vi "Range.vi"(8 "Exponent":dbl=1.0, 9 "End":dbl, 10 "Start":dbl, 11 "Steps":i32) -> (3 "Array":dbl[](array[numeric]))   [LabVIEW 2017]
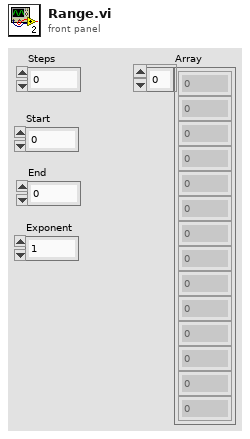
[diagram p1: front panel]
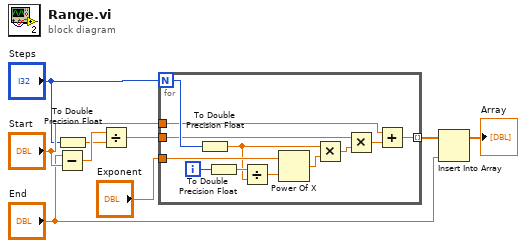
[diagram p0: block diagram]
diagram:
  n1 = Subtract(x="End", y="Start") -> (x-y=w9:dbl)
  n2 = To Double Precision Float(number="Steps") -> (double precision float=w8:dbl)
  n3 = Divide(x=w9, y=w8) -> (x/y=w6:dbl)
  n4 = for {
    N: "Steps" -> [w19]
    tunnel: [w10] -> w3 mode=indexing
    tunnel: "Exponent" -> [w17]
    tunnel: w6 -> [w14]
    tunnel: "Start" -> [w13]
    i -> [w21]
    n5 = To Double Precision Float(number=w19) -> (double precision float=w16:dbl)
    n6 = To Double Precision Float(number=w21) -> (double precision float=w20:dbl)
    n7 = Divide(x=w20, y=w16) -> (x/y=w18:dbl)
    n8 = Power Of X(1:w18, 2:w17) -> (0:w15:dbl)
    n9 = Multiply(x=w16, y=w15) -> (x*y=w11:dbl)
    n10 = Multiply(x=w14, y=w11) -> (x*y=w12:dbl)
    n11 = Add(x=w13, y=w12) -> (x+y=w10:dbl)
  }
  n12 = Insert Into Array(array=w3, new element="End") -> (→"Array":dbl[])  [unwired: 1 in]
